vi "Manual_mode.vi"(8 "error in (no error)":errorcluster) -> (0 "error in (out)":errorcluster)   [LabVIEW 2024, in "MANUAL_MODE.lvlib"]
doc: "This template is for the Queued Message Handler design pattern.\n\nThe Event Handling Loop generates messages based on user interface actions.\n\nThe Message Handling Loop processes messages generated by the Event Handling Loop, or by other messages. The messages are string values, so new messages can be added easily to the Message Cases case structure in the Message Handling Loop. Each message cluster can also provide an optional value for Message Data, which is a variant that can be converted to whatever message-specific data is required."
uses:
  MANUAL_MODE.lvlib
  support/FCT_DO_UI.ctl
  support/EOL_DO_UI.ctl
  controls/Manual UI Data.ctl
  PrivateControls/FGV_Queue_Control.ctl
  ADAM_DI/support/Relay_enum_IN.ctl
  <vilib>/Utility/error.llb/Error Cluster From Error Code.vi
  <vilib>/ErrorRing/Error Ring.xnode
  support/Message Queue/Manual Message Queue.lvlib
  support/User Event - Stop/Manual User Event - Stop.lvlib
  Launcher/Launcher_DTU.lvlib
  ADAM_DI/ADAM_DI.lvlib
  Relay_Module/Relay_Module.lvlib
panel:
  in  "Tab Control":T1(tab)
  in  "FCT/EOL":u16(ring) items=["<SELECT>", "FCT", "EOL"]
  in  "Init. INSTR.":bool
  in  "Exit":bool
  in  "DUT":u8=1 min=1 max=10 step=1
  in  "Relay-FCT/EOL":enum32{"FCT", "EOL"}(tab)
  in  "FCT_Relay - OUTPUT":T2
  in  "EOL_Relay - OUTPUT":T3
  out "ADAM_Card - INPUT":T4
  out "queue name 2":string
  out "queue name":string
  out "Display <Replace Me>":string
  # "These controls have associated \"Value Changed\" events configured in the Event Structure on the diagram.\n\nReplace them (and reconfigure the Event Structure) with the controls you need for your application."
  # "This template is for the Queued Message Handler design pattern.\n\nSee the block diagram for more information on how to use this template."
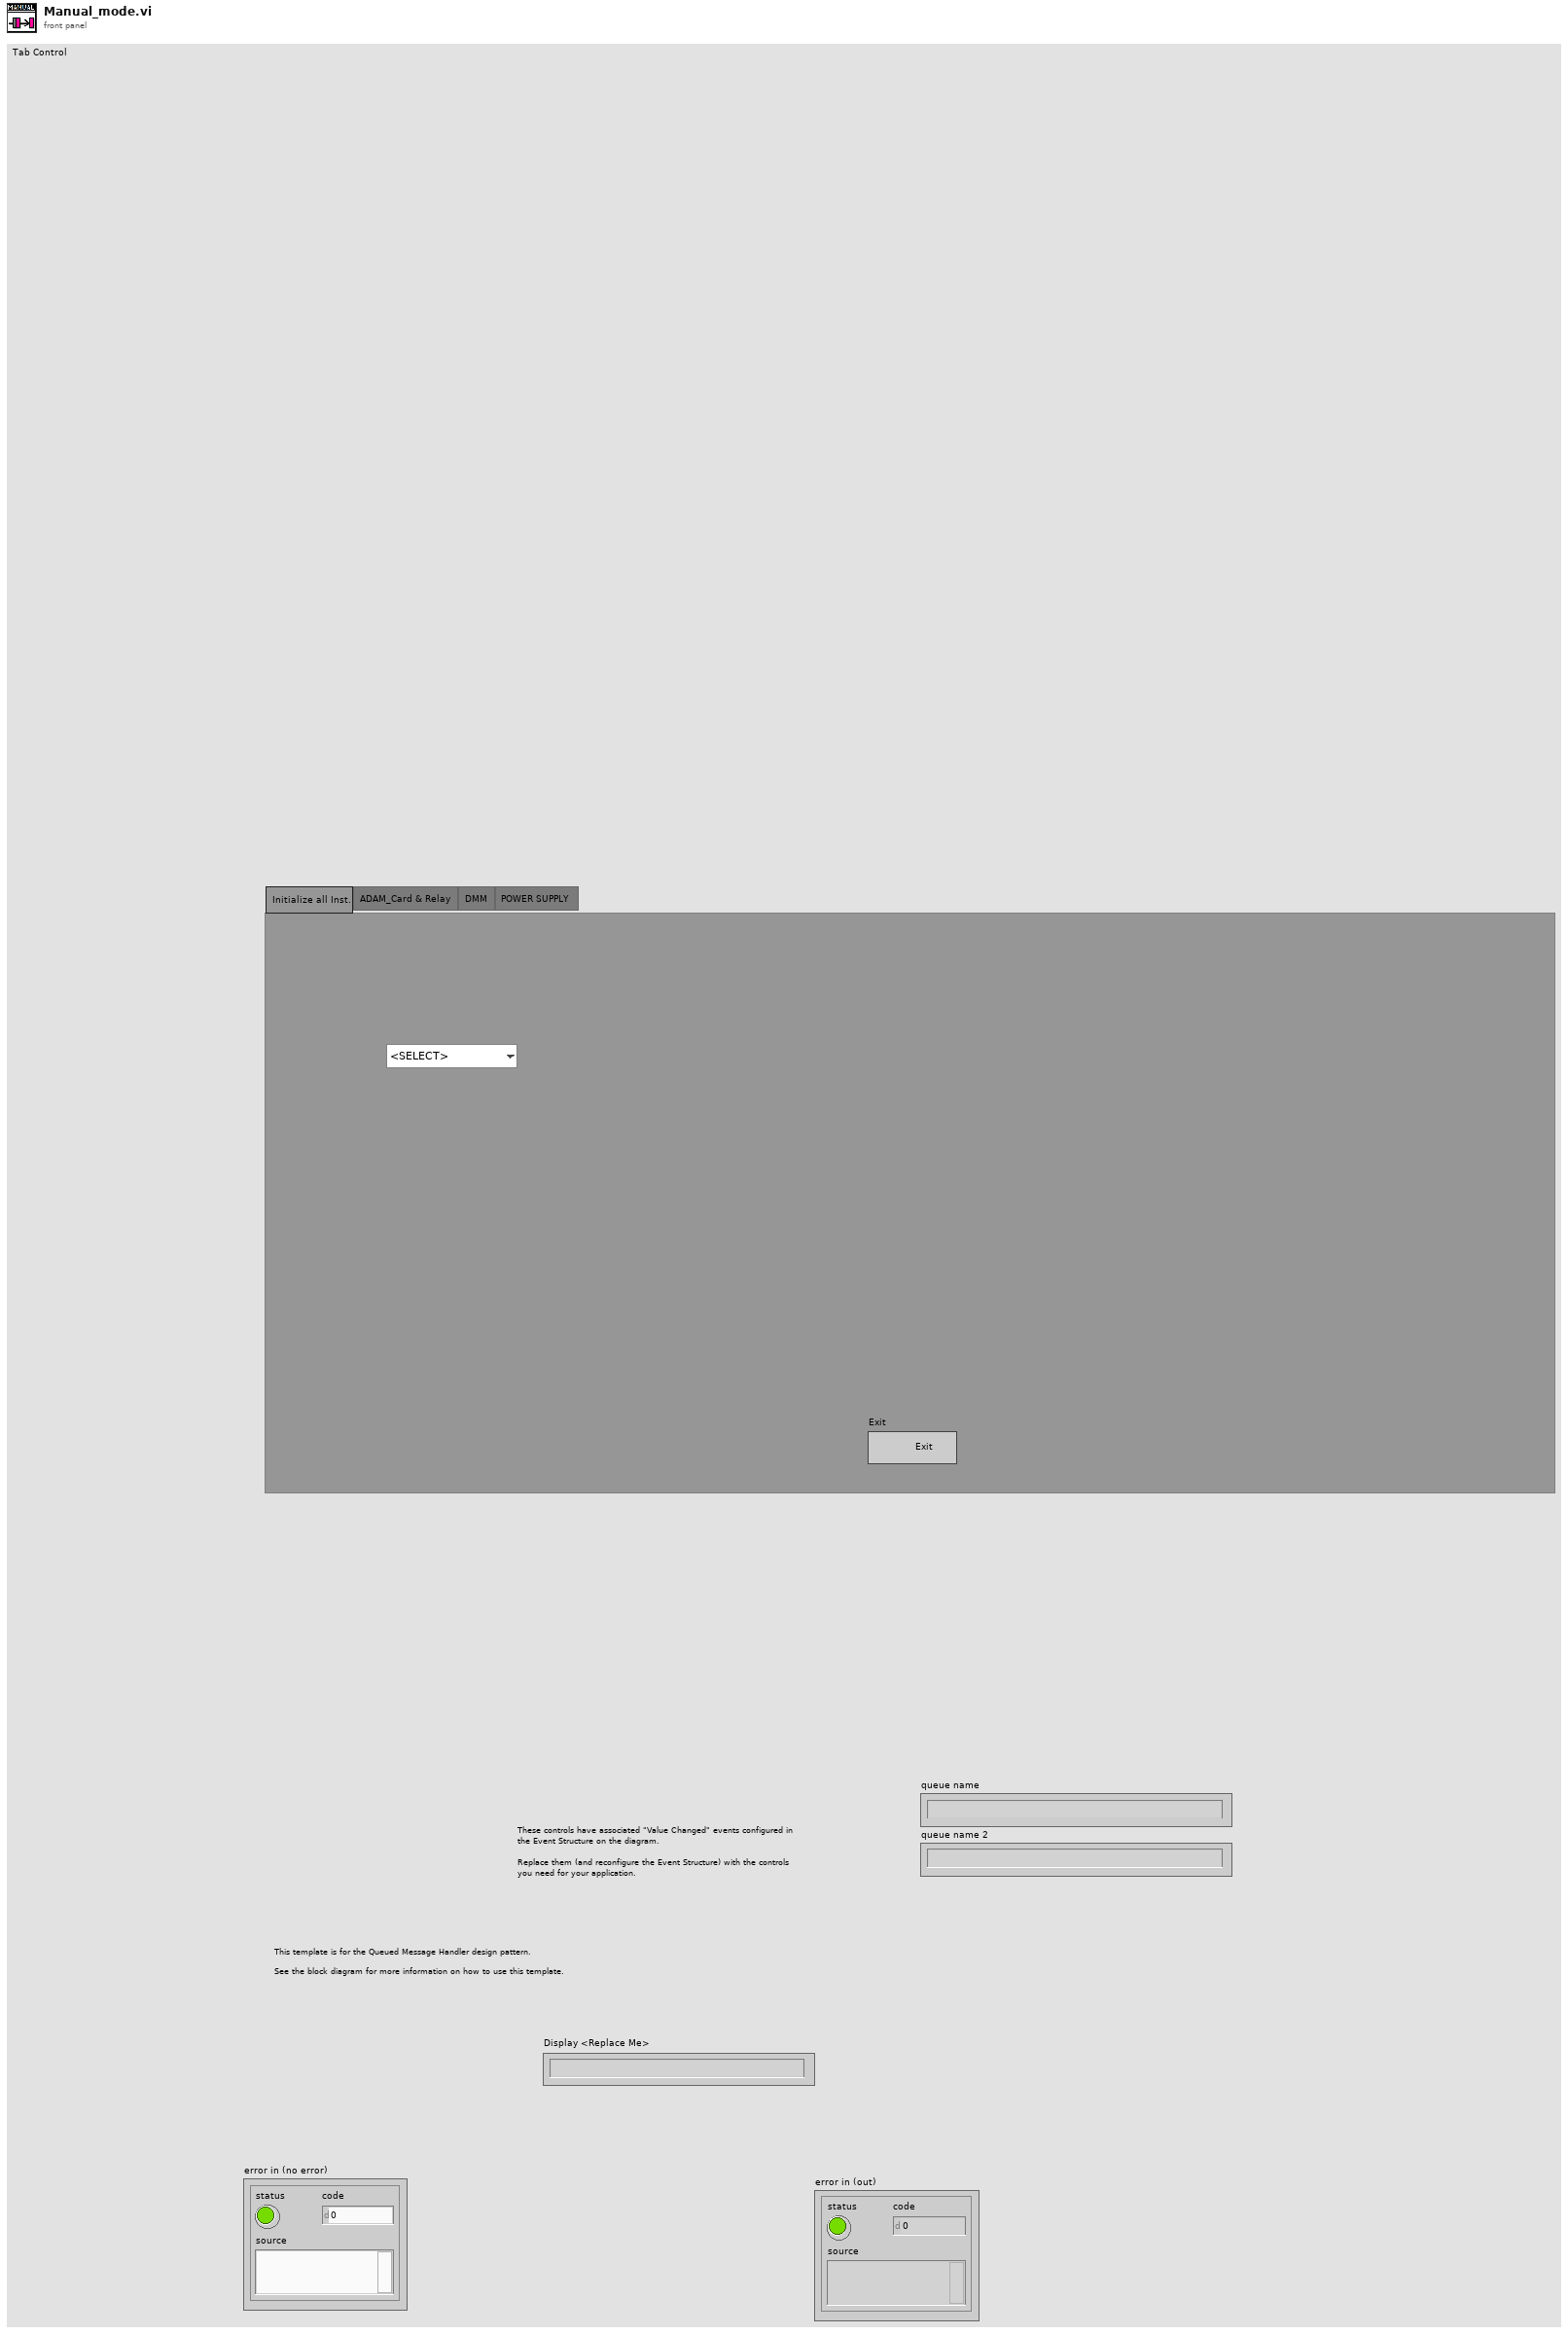
[diagram p1: front panel]
types:
  T1 = enum32{"Initialize all Inst.", "ADAM_Card & Relay", "DMM", "POWER SUPPLY"}
  T2 = typedef "FCT_DO_UI.ctl" = cluster{"CONN_SUPPLY":bool, "HB_CONN":bool, "L_IND_CONN":bool, "R_IND_CONN":bool, "SW1":bool, "SW2":bool, "CAN_H":bool, "CAN_L":bool, "CYLINDER_ON/OFF":bool, "SPARE_1":bool, "SPARE_2":bool, "Tower Red":bool, "Tower Amber":bool, "Tower Green":bool, "Tower Buzzer":bool, "SLIMRELAY_DUT":bool}
  T3 = typedef "EOL_DO_UI.ctl" = cluster{"GND_DMM":bool, "CAN_H_RES":bool, "CAN_L_RES":bool, "L_IND_RES":bool, "R_IND_RES":bool, "HB_CONN_DMM":bool, "14V_RES":bool, "CAN_L_(DMM-)":bool, "CAN_H":bool, "CAN_L":bool, "14V":bool, "GND":bool, "HB_CONN":bool, "L_IND":bool, "R_IND":bool, "CYLINDER_DUT":bool, "CYL_PB_1":bool, "CYL_PB_2":bool, "DUT_PASS":bool, "DUT_FAIL":bool, "SPARE1":bool, "Tower Red_EOL":bool, "Tower Amber_EOL":bool, "Tower Green_EOL":bool, "Tower Buzzer_EOL":bool}
  T4 = cluster{"EMERGENCY":bool, "CONTROL ON":bool, "START DUT 1":bool, "START DUT 2":bool, "STOP DUT 1":bool, "STOP DUT 2":bool, "FCT PPS 1":bool, "FCT PPS 2":bool, "DUT 1 REED CYL UP":bool, "DUT 1 REED CYL DOWN":bool, "DUT 2 REED CYL UP":bool, "DUT 2 REED CYL DOWN":bool, "LIGHT CURTAIN":bool}
  T5 = typedef "MANUAL_MODE.lvlib/FGV_Queue_Control.ctl" = enum16{"Release", "Get", "Set"}
  T6 = typedef "MANUAL_MODE.lvlib/Manual UI Data.ctl" = cluster{"Boolean <Replace Me>":bool, "Status":string, "Numeric <Replace Me>":dbl, "Configuration_Path":path, "Equipment_Combined_Path":path, "Equipment_Common_Path":path, "Equip_List_Common":string[], "Equip_List_Combined":string[], "DTU1_Common-Array_Q":refnum<queue>[], "DTU2_Common-Array_Q":refnum<queue>[], "DTU1_Combined-Array_Q":refnum<queue>[], "DTU2_Combined-Array_Q":refnum<queue>[], "DTU1_Common-Array_N":refnum<notifier>[], "DTU2_Common-Array_N":refnum<notifier>[], "DTU1_Combined-Array_N":refnum<notifier>[], "DTU2_Combined-Array_N":refnum<notifier>[], "ADAM_loop_Q":refnum<queue>, "DUT":u8, "FCT/EOL":u16}
  T7 = typedef "MANUAL_MODE.lvlib/Manual Message Queue.lvlib/All Message Queues.ctl" = cluster{"UI":refnum<queue>, "QSM":refnum<queue>}
  T8 = cluster{"Message":string, "Message Data":variant}
  T9 = enum16{"Read", "Write", "All_sections", "All_values", "Remove key&section"}
  T10 = typedef "Relay_Module.lvlib/Relay_Enum_OUT.ctl" = enum16{"CONN_SUPPLY_%d_FCT", "HB_CONN_%d_FCT", "L_IND_CONN_%d_FCT", "R_IND_CONN_%d_FCT", "SW1_%d_FCT", "SW2_%d_FCT", "CAN_H_%d_FCT", "CAN_L_%d_FCT", "CYLINDER_ON/OFF_%d_FCT", "SPARE_1_%d_FCT", "SPARE_2_%d_FCT", "Tower Red", "Tower Amber", "Tower Green", "Tower Buzzer", "SLIMRELAY_DUT_%d_FCT", "GND_DMM_%d_EOL", "CAN_H_RES_%d_EOL", "CAN_L_RES_%d_EOL", "L_IND_RES_%d_EOL", "R_IND_RES_%d_EOL", "HB_CONN_DMM_%d_EOL", "14V_RES_%d_EOL", "CAN_L_(DMM-)_%d_EOL", "CAN_H_%d_EOL", "CAN_L_%d_EOL", "14V_%d_EOL", "GND_%d_EOL", "HB_CONN_%d_EOL", "L_IND_%d_EOL", "R_IND_%d_EOL", "CYLINDER_DUT_%d_EOL", "CYL_PB_1_%d_EOL", "CYL_PB_2_%d_EOL", "DUT_PASS_%d_EOL", "DUT_FAIL_%d_EOL", "SPARE1_%d_EOL", "Tower Red_EOL", "Tower Amber_EOL", "Tower Green_EOL", "Tower Buzzer_EOL"}
  T11 = typedef "ADAM_DI.lvlib/Relay_enum_IN.ctl" = enum16{"EMERGENCY", "CONTROL ON", "START DUT 1", "START DUT 2", "STOP DUT 1", "STOP DUT 2", "PPS DUT 1", "PPS DUT 2", "REED CYL UP DUT 1", "REED CYL DOWN DUT 1", "REED CYL UP DUT 2", "REED CYL DOWN DUT 2", "LIGHT CURTAIN"}
  T12 = cluster{"DOs_out[0]":bool, "DOs_out[1]":bool, "DOs_out[2]":bool, "DOs_out[3]":bool, "DOs_out[4]":bool, "DOs_out[5]":bool, "DOs_out[6]":bool, "DOs_out[7]":bool, "DOs_out[8]":bool, "DOs_out[9]":bool, "DOs_out[10]":bool, "DOs_out[11]":bool, "DOs_out[12]":bool}
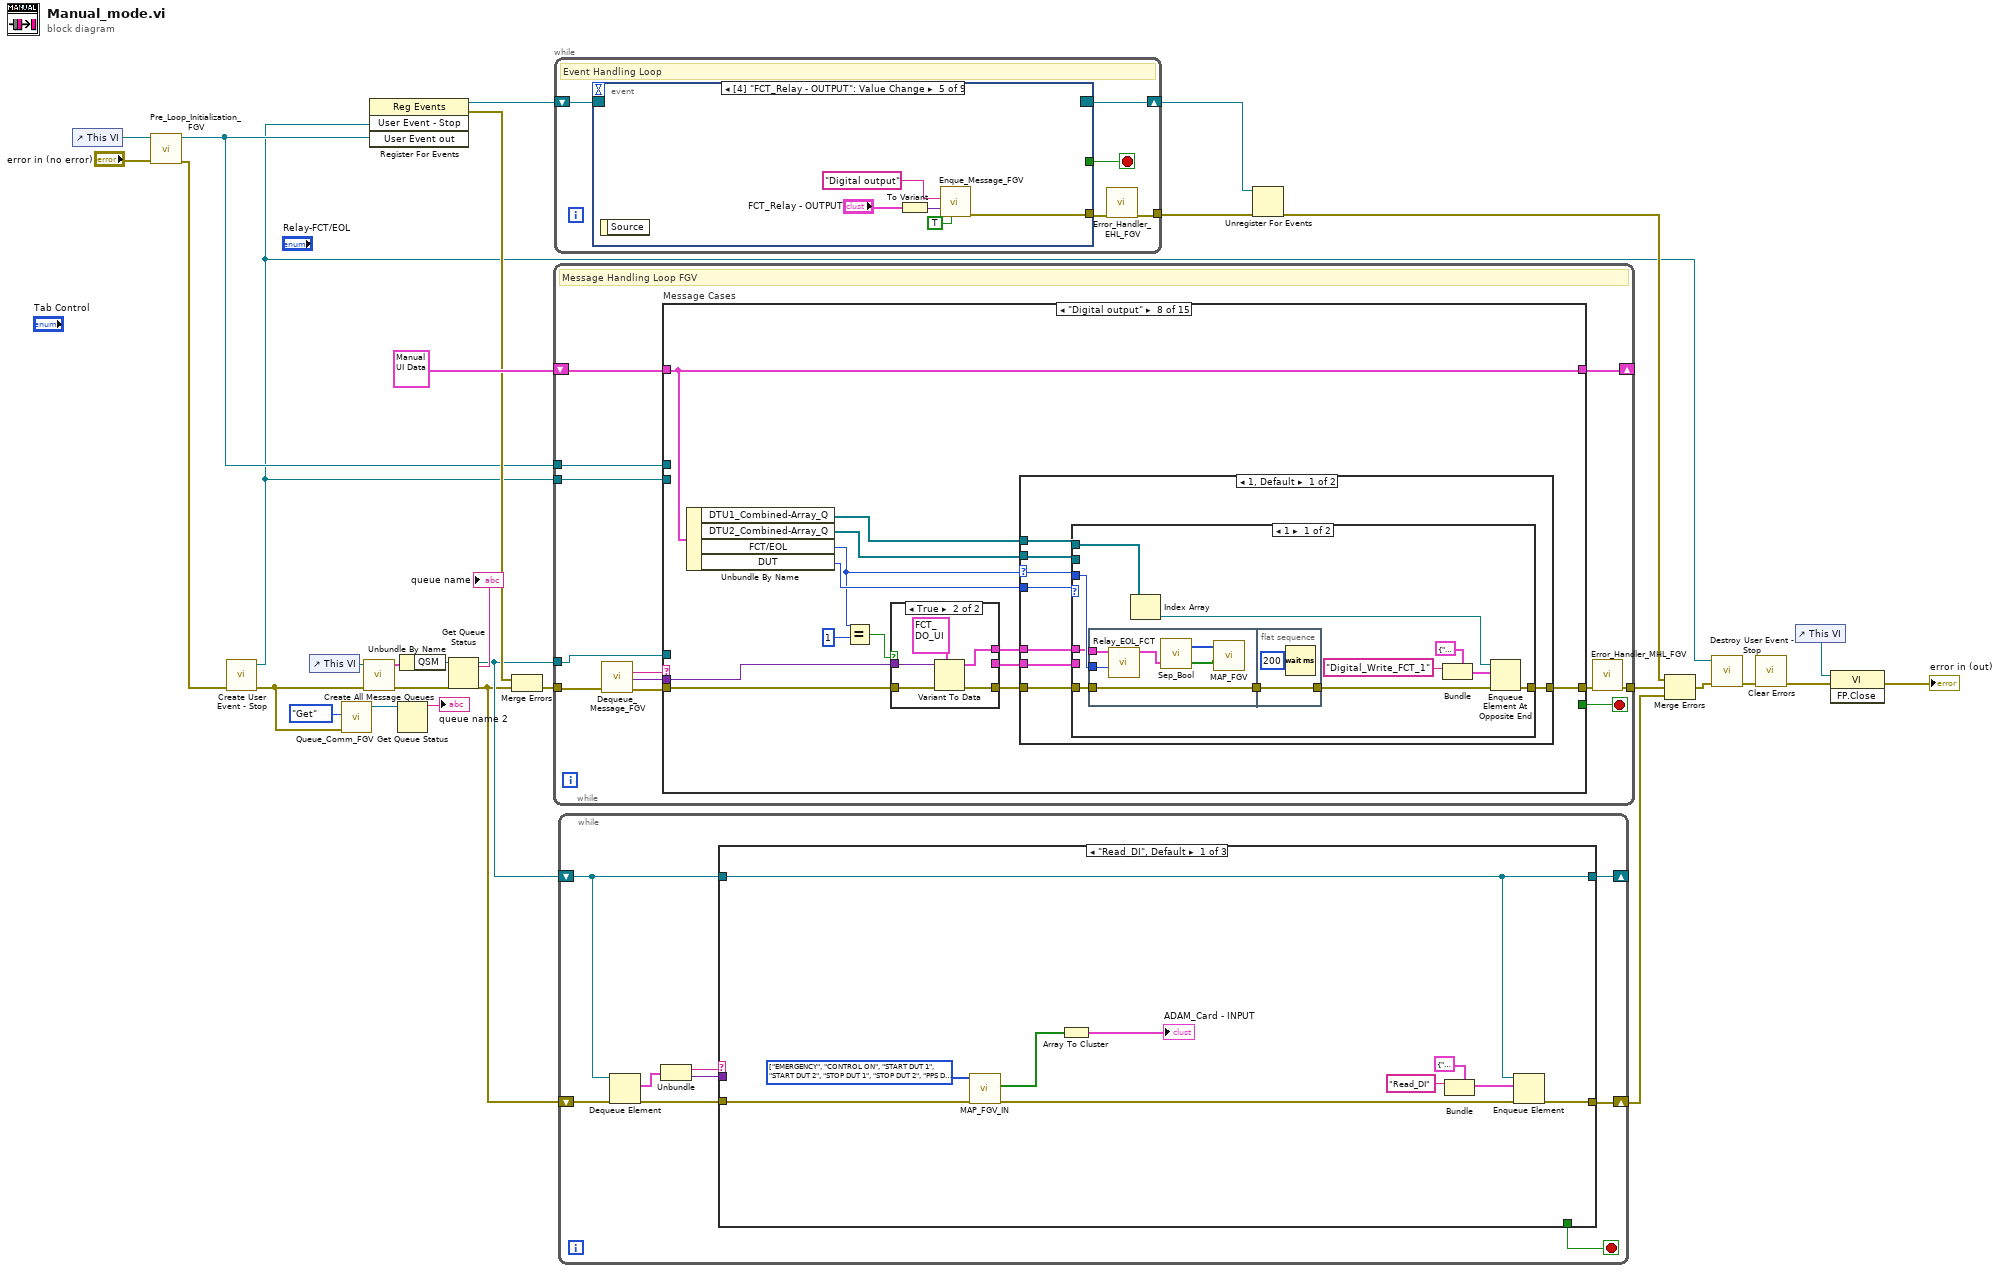
[diagram p0: block diagram]
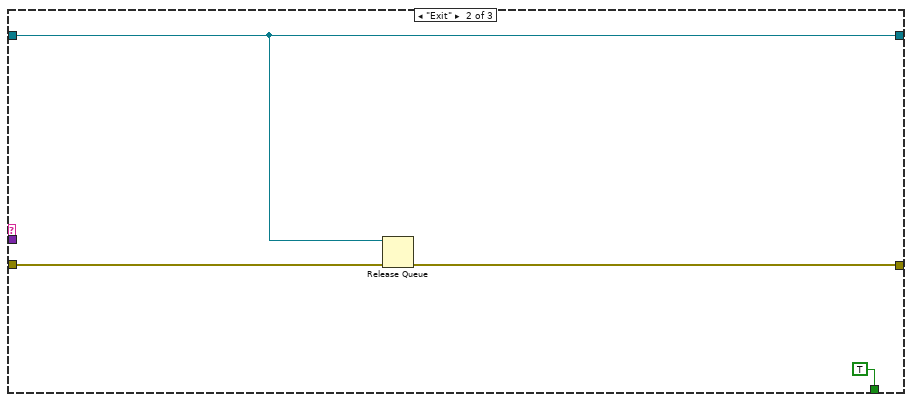
[diagram p2: hidden frame]
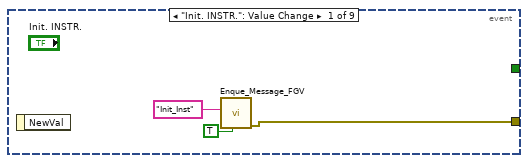
[diagram p4: hidden frame]
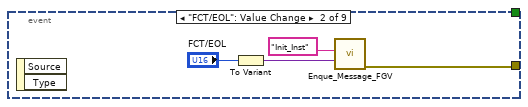
[diagram p5: hidden frame]
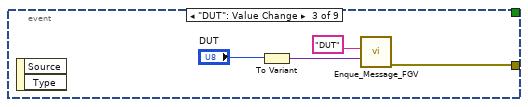
[diagram p6: hidden frame]
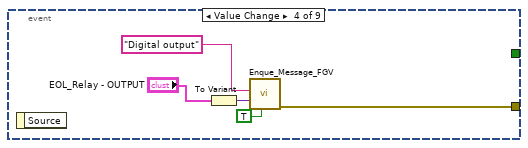
[diagram p7: hidden frame]
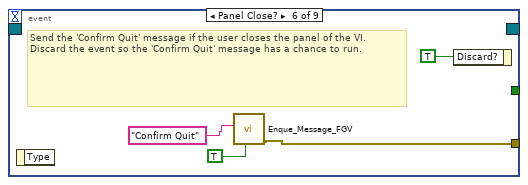
[diagram p8: hidden frame]
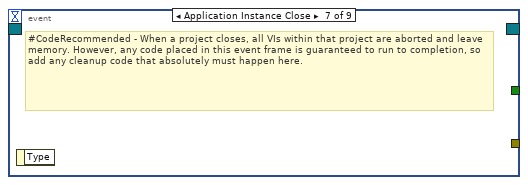
[diagram p9: hidden frame]
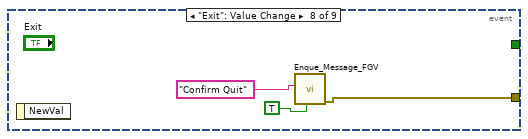
[diagram p10: hidden frame]
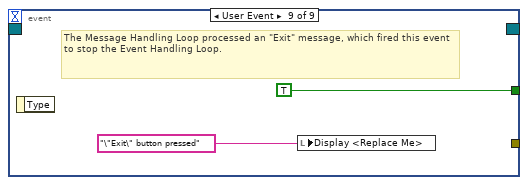
[diagram p11: hidden frame]
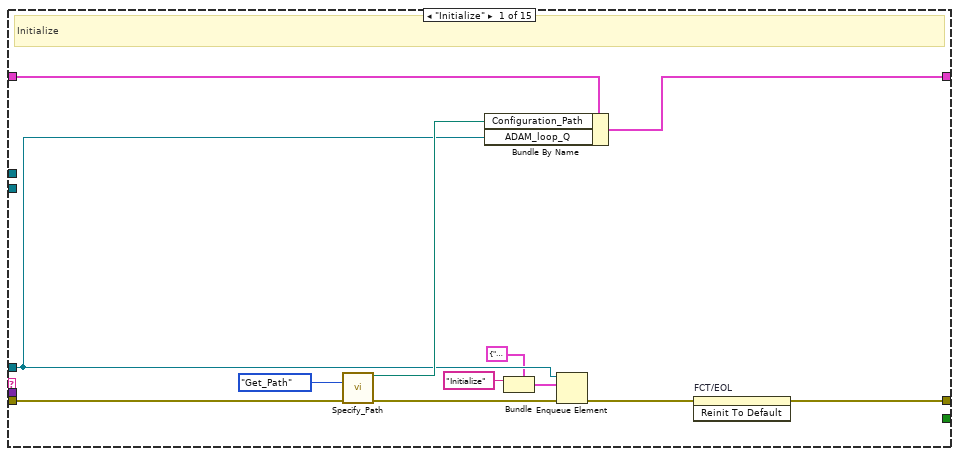
[diagram p12: hidden frame]
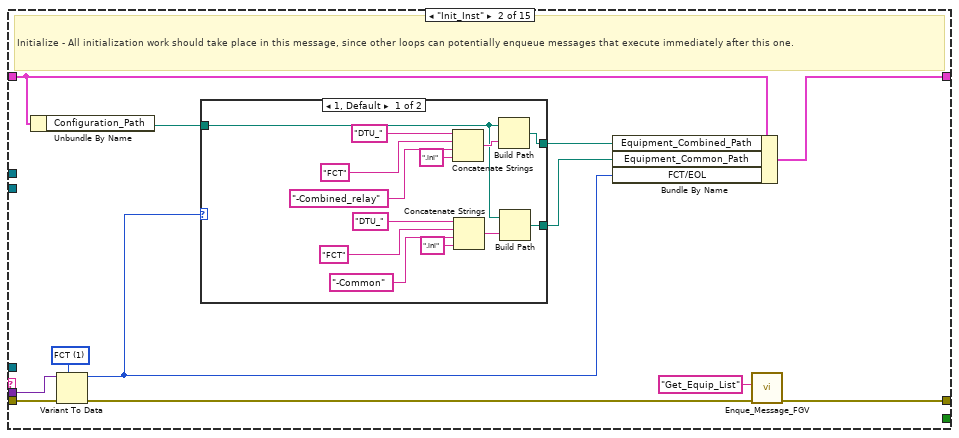
[diagram p13: hidden frame]
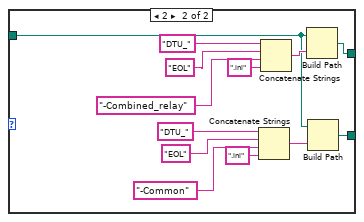
[diagram p14: hidden frame]
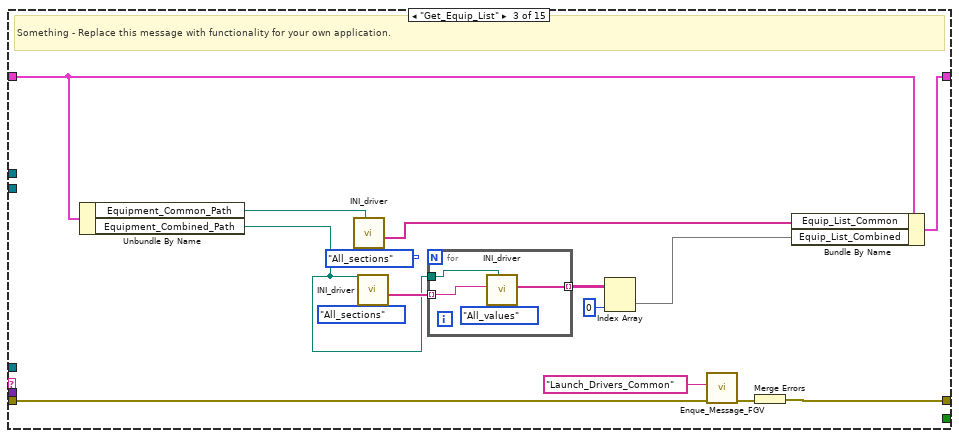
[diagram p15: hidden frame]
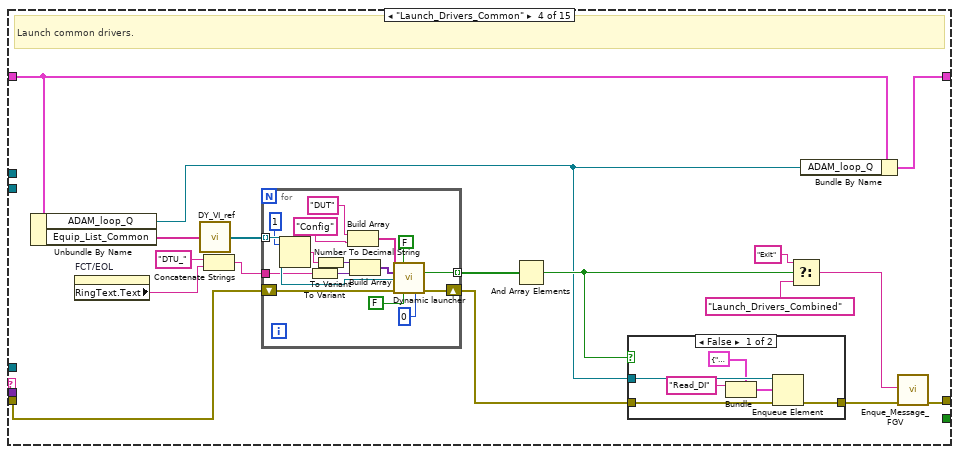
[diagram p16: hidden frame]
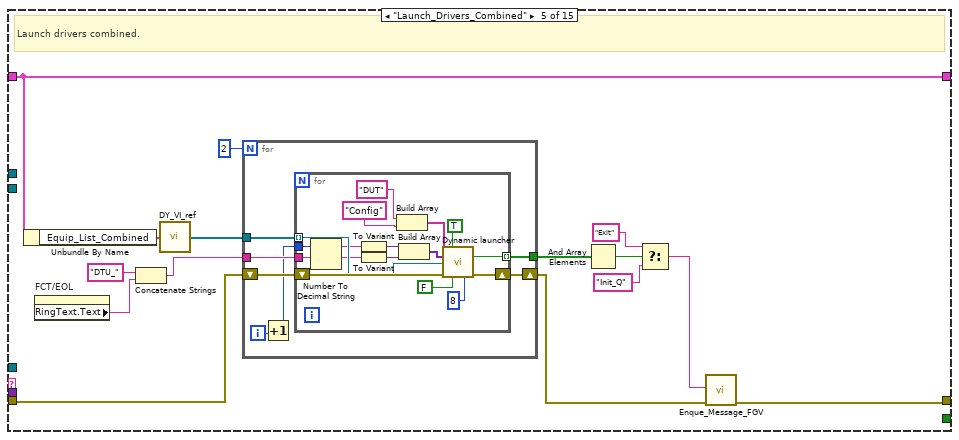
[diagram p18: hidden frame]
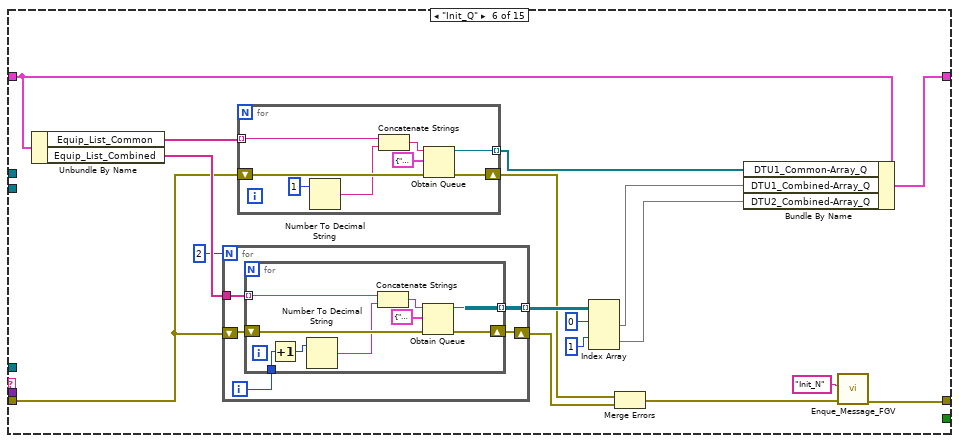
[diagram p19: hidden frame]
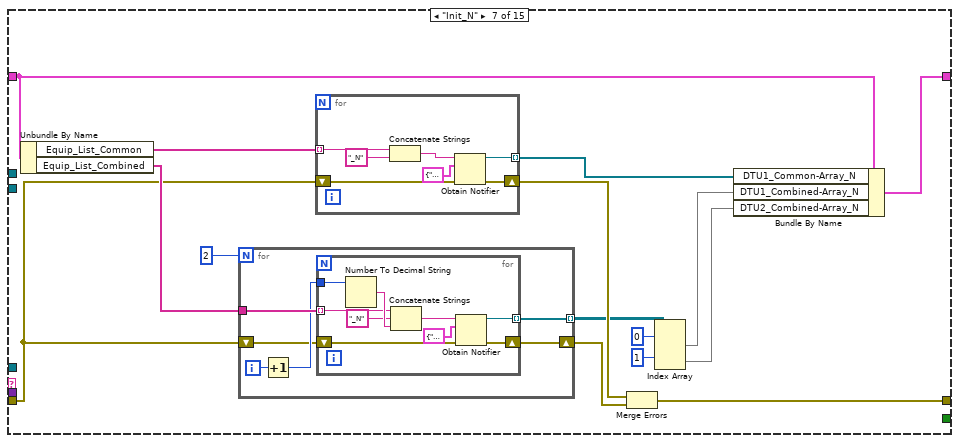
[diagram p20: hidden frame]
diagram:
  n1 = control-ref of="This VI"() -> (w18:refnum<vi>)
  n2 = call "Pre_Loop_Initialization_FGV.vi"("error in (no error)"="error in (no error)", "VI in"=w18) -> ("error out"=w16:errorcluster, "User Event out"=w8:refnum<user-event>)  [unwired: 8 in]
  n3 = call "Create User Event - Stop.vi"("error in (no error)"=w16) -> ("error out"=w12:errorcluster, "User Event - Stop"=w7:refnum<user-event>)  [unwired: 9 in]
  n4 = control-ref of="This VI"() -> (w14:refnum<vi>)
  n5 = call "Queue_Comm_FGV.vi"("error in (no error)"=w12, "Enum"=FGV_Queue_Control."Get") -> ("queue Out"=w10:refnum<queue>)  [unwired: 8 in, 1 out]
  n6 = call "Create All Message Queues.vi"("error in (no error)"=w12, "This VI"=w14) -> ("error out"=w5:errorcluster, "Message Queues out"=w29:T7)  [unwired: 8 in]
  n7 = register-events(w7, w8) -> (reference out=w21:refnum<event-registration>, error out=w19:errorcluster)  [unwired: 2 in]
  n8 = Get Queue Status(queue=w10) -> (queue name=→"queue name 2":string)  [unwired: 2 in, 7 out]
  n9 = Unbundle By Name(w29) -> ("QSM"=w27:refnum<queue>)
  n10 = Get Queue Status(queue=w27) -> (queue out=w6:refnum<queue>, queue name=→"queue name":string)  [unwired: 2 in, 6 out]
  n11 = Merge Errors(w19, w5) -> (w20:errorcluster)
  n12 = while {
    tunnel: w6 -> [w30]
    shift-right: [w40] -> _
    shift-left: T6 {"Boolean <Replace Me>"=FALSE, "Status"="", "Numeric <Replace Me>"=0.0, "Configuration_Path"=path "", "Equipment_Combined_Path"=path "", "Equipment_Common_Path"=path "", "Equip_List_Common"=[], "Equip_List_Combined"=[], "DTU1_Common-Array_Q"=[], "DTU2_Common-Array_Q"=[], "DTU1_Combined-Array_Q"=[], "DTU2_Combined-Array_Q"=[], "DTU1_Common-Array_N"=[], "DTU2_Common-Array_N"=[], "DTU1_Combined-Array_N"=[], "DTU2_Combined-Array_N"=[], "ADAM_loop_Q"=refnum, "DUT"=1, "FCT/EOL"=0} ("Data Cluster") -> [w41]
    tunnel: w8 -> [w38]
    tunnel: w20 -> [w37]
    tunnel: [w32] -> w28
    tunnel: w7 -> [w31]
    stop <- w39 stop-if-true
    # "Message Handling Loop FGV"
    n13 = call "Dequeue_Message_FGV.vi"("error in (no error)"=w37) -> ("error out"=w36:errorcluster, "Message Data"=w35:variant, "Message"=w34:string)  [unwired: 8 in]
    n14 = case "Message Cases" shown="\"Digital output\"" w34 {
      selector: w34 -> [_ _ _ _ _ _ _ _ _ _ _ _ _ _ w499]
      tunnel: w36 -> [w49 w64 w104 w119 w156 w195 w239 w277 w387 w392 w401 w411 w445 w484 _]
      tunnel: [w42 w65 w106 w127 w165 w191 w236 w275 w384 w393 w395 w419 w453 w493 w500] -> w33
      tunnel: w41 -> [w52 w62 w103 w126 w164 w199 w230 w276 w386 w394 w400 w409 w452 w495 w501]
      tunnel: [w51 w59 w102 w115 w164 w198 w229 w276 w385 w394 w400 w409 w452 w495 w501] -> w40
      tunnel: [_ _ _ _ _ _ _ _ _ _ _ _ _ TRUE _] -> w39
      tunnel: w35 -> [_ w57 _ _ _ _ _ w270 w383 w391 w399 _ _ w491 _]
      tunnel: w38 -> [_ _ _ _ _ _ _ _ _ _ _ _ _ w492 _]
      tunnel: w31 -> [_ _ _ _ _ _ _ _ _ _ _ _ _ w488 _]
      tunnel: w30 -> [w47 _ _ _ _ _ _ _ _ _ _ w412 _ _ _]
      frame "Initialize" {
        # "Initialize"
        n15 = call "Specify_Path.vi"("Path_Enum"=enum16{"Find_Path", "Get_Path"}."Get_Path", "error in (no error)"=w49) -> ("Configurations"=w50:path, "error out"=w48:errorcluster)  [unwired: 6 in, 6 out]
        n16 = Bundle By Name(cluster=w52, "Configuration_Path"=w50, "ADAM_loop_Q"=w47) -> (w51:T6)
        n17 = Bundle(cluster=T8 {"Message"="", "Message Data"=variant} ("Message Cluster"), "Message"="Initialize") -> (w45:T8)  [unwired: 1 in]
        n18 = Enqueue Element(queue=w47, element=w45, error in (no error)=w48) -> (error out=w43:errorcluster)  [unwired: 1 in, 2 out]
        n19 = invoke on="FCT/EOL" class="Ring (strict)" method="Reinit To Default"(error in=w43) -> (error out=w42:errorcluster)  [unwired: 2 in, 2 out]
      }
      frame "Init_Inst" {
        w54 = u16 1 items=["<SELECT>", "FCT", "EOL"] ("FCT/EOL")
        # "Initialize - All initialization work should take place in this message, since other loops can potentially enqueue messages that execute immediately after this one."
        n20 = Unbundle By Name(w62) -> ("Configuration_Path"=w63:path)
        n21 = Variant To Data(error in=w64, type=w54, Variant=w57) -> (data=w55:u16, error out=w58:errorcluster)
        n22 = case shown="1, Default" w55 {
          tunnel: w63 -> [w66 w82]
          tunnel: [w68 w81] -> w61
          tunnel: [w67 w80] -> w60
          frame 1, Default {
            n23 = Concatenate Strings("DTU_" ("string"), "FCT" ("regular expression"), "-Combined_relay" ("string"), ".ini" ("string")) -> (w78:string)
            n24 = Concatenate Strings("DTU_" ("string"), "FCT" ("regular expression"), "-Common" ("string"), ".ini" ("string")) -> (w69:string)
            n25 = Build Path(base path=w66, name or relative path=w78) -> (appended path=w68:path)
            n26 = Build Path(base path=w66, name or relative path=w69) -> (appended path=w67:path)
          }
          frame 2 {
            n27 = Concatenate Strings("DTU_" ("string"), "EOL" ("regular expression"), "-Common" ("string"), ".ini" ("string")) -> (w83:string)
            n28 = Concatenate Strings("DTU_" ("string"), "EOL" ("regular expression"), "-Combined_relay" ("string"), ".ini" ("string")) -> (w91:string)
            n29 = Build Path(base path=w82, name or relative path=w91) -> (appended path=w81:path)
            n30 = Build Path(base path=w82, name or relative path=w83) -> (appended path=w80:path)
          }
        }
        n31 = Bundle By Name(cluster=w62, "Equipment_Combined_Path"=w61, "Equipment_Common_Path"=w60, "FCT/EOL"=w55) -> (w59:T6)
        n32 = call "Enque_Message_FGV.vi"("error in (no error)"=w58, "Message"="Get_Equip_List") -> ("error out"=w65:errorcluster)  [unwired: 9 in]
      }
      frame "Get_Equip_List" {
        # "Something - Replace this message with functionality for your own application."
        n33 = Unbundle By Name(w103) -> ("Equipment_Common_Path"=w97:path, "Equipment_Combined_Path"=w96:path)
        n34 = call "INI_driver.vi"("Enum"=T9."All_sections", "instrument file path"=w97) -> ("section names"=w92:string[])  [unwired: 6 in, 3 out]
        n35 = call "INI_driver.vi"("Enum"=T9."All_sections", "instrument file path"=w96) -> ("section names"=w98:string[])  [unwired: 6 in, 3 out]
        n36 = for {
          tunnel: w98 -> [w110] mode=indexing
          tunnel: w96 -> [w109]
          tunnel: [w107] -> w94 mode=indexing
          n37 = call "INI_driver.vi"("Enum"=T9."All_values", "instrument file path"=w109, "Section"=w110) -> ("Values out"=w107:string[])  [unwired: 5 in, 3 out]
        }
        n38 = Index Array(array=w94, index (col)=0 ("disabled index (col)")) -> (element=w93:string[])  [unwired: 1 in]
        n39 = call "Enque_Message_FGV.vi"("error in (no error)"=w104, "Message"="Launch_Drivers_Common") -> ("error out"=w105:errorcluster)  [unwired: 9 in]
        n40 = Merge Errors(w105) -> (w106:errorcluster)
        n41 = Bundle By Name(cluster=w103, "Equip_List_Common"=w92, "Equip_List_Combined"=w93) -> (w102:T6)
      }
      frame "Launch_Drivers_Common" {
        # "Launch common drivers."
        n42 = Unbundle By Name(w126) -> ("ADAM_loop_Q"=w114:refnum<queue>, "Equip_List_Common"=w125:string[])
        n43 = property on="FCT/EOL" class="Ring (strict)"() -> ("RingText.Text"=w112:string)  [unwired: 2 in, 2 out]
        n44 = call "DY_VI_ref.vi"("EQUIP LIST"=w125) -> ("VI_ref"=w124:refnum<vi>[])
        n45 = Concatenate Strings("DTU_", w112) -> (w111:string)
        n46 = for {
          shift-right: [w150] -> w118
          shift-left: w119 -> [w142]
          tunnel: [w149] -> w122 mode=indexing
          tunnel: w124 -> [w138] mode=indexing
          tunnel: w111 -> [w137]
          n47 = Number To Decimal String(number=1) -> (decimal integer string=w135:string)  [unwired: 1 in]
          n48 = To Variant(anything=w137) -> (Variant=w143:variant)
          n49 = To Variant(anything=w135) -> (Variant=w144:variant)
          n50 = Build Array("DUT", "Config") -> (w146:string[])
          n51 = Build Array(w144, w143) -> (w145:variant[])
          n52 = call "Dynamic launcher.vi"("element"=w146, "Clone ?"=FALSE, "Value"=w145, "VI Refnum"=w138, "error in (no error)"=w142, "Open FP"=FALSE, "options"=0) -> ("Failed"=w149:bool, "error out"=w150:errorcluster)  [unwired: 6 in, 1 out]
        }
        n53 = And Array Elements(Boolean array=w122) -> (logical AND=w116:bool)
        n54 = case shown="False" w116 {
          tunnel: w118 -> [w133 w134]
          tunnel: [w132 w134] -> w117
          tunnel: w114 -> [w131 _]
          frame False {
            n55 = Bundle(cluster=T8 {"Message"="", "Message Data"=variant} ("Message Cluster"), "Message"="Read_DI") -> (w128:T8)  [unwired: 1 in]
            n56 = Enqueue Element(queue=w131, element=w128, error in (no error)=w133) -> (error out=w132:errorcluster)  [unwired: 1 in, 2 out]
          }
          frame True {
          }
        }
        n57 = Select(t="Exit" ("f"), s=w116, f="Launch_Drivers_Combined") -> (s? t:f=w120:string)
        n58 = Bundle By Name(cluster=w126, "ADAM_loop_Q"=w114) -> (w115:T6)
        n59 = call "Enque_Message_FGV.vi"("error in (no error)"=w117, "Message"=w120) -> ("error out"=w127:errorcluster)  [unwired: 9 in]
      }
      frame "Launch_Drivers_Combined" {
        # "Launch drivers combined."
        n60 = Unbundle By Name(w164) -> ("Equip_List_Combined"=w163:string[])
        n61 = property on="FCT/EOL" class="Ring (strict)"() -> ("RingText.Text"=w152:string)  [unwired: 2 in, 2 out]
        n62 = Concatenate Strings("DTU_", w152) -> (w151:string)
        n63 = call "DY_VI_ref.vi"("EQUIP LIST"=w163) -> ("VI_ref"=w162:refnum<vi>[])
        n64 = for {
          N: 2 -> [_]
          tunnel: w162 -> [w172]
          tunnel: [w171] -> w159
          shift-right: [w169] -> w155
          shift-left: w156 -> [w170]
          tunnel: w151 -> [w167]
          i -> [w168]
          n65 = Increment(x=w168) -> (x+1=w166:i32)
          n66 = for {
            shift-right: [w188] -> w169
            shift-left: w170 -> [w180]
            tunnel: [w187] -> w171 mode=indexing
            tunnel: w172 -> [w176] mode=indexing
            tunnel: w166 -> [w175]
            tunnel: w167 -> [w174]
            n67 = Number To Decimal String(number=w175) -> (decimal integer string=w173:string)  [unwired: 1 in]
            n68 = To Variant(anything=w173) -> (Variant=w182:variant)
            n69 = To Variant(anything=w174) -> (Variant=w181:variant)
            n70 = Build Array("DUT", "Config") -> (w184:string[])
            n71 = Build Array(w182, w181) -> (w183:variant[])
            n72 = call "Dynamic launcher.vi"("element"=w184, "Clone ?"=TRUE, "Value"=w183, "VI Refnum"=w176, "error in (no error)"=w180, "Open FP"=FALSE, "options"=8) -> ("Failed"=w187:bool, "error out"=w188:errorcluster)  [unwired: 6 in, 1 out]
          }
        }
        n73 = And Array Elements(Boolean array=w159) -> (logical AND=w160:bool)
        n74 = Select(t="Exit" ("f"), s=w160, f="Init_Q") -> (s? t:f=w157:string)
        n75 = call "Enque_Message_FGV.vi"("error in (no error)"=w155, "Message"=w157) -> ("error out"=w165:errorcluster)  [unwired: 9 in]
      }
      frame "Init_Q" {
        n76 = Unbundle By Name(w199) -> ("Equip_List_Common"=w205:string[], "Equip_List_Combined"=w204:string[])
        n77 = for {
          N: 2 -> [_]
          tunnel: w204 -> [w218]
          tunnel: [w216] -> w201 mode=indexing
          shift-right: [w214] -> w193
          shift-left: w195 -> [w215]
          i -> [w217]
          n78 = for {
            shift-right: [w226] -> w214
            shift-left: w215 -> [w227]
            tunnel: w218 -> [w223] mode=indexing
            tunnel: [w222] -> w216 mode=indexing
            tunnel: w217 -> [w219]
            n79 = Increment(x=w219) -> (x+1=w220:i32)
            n80 = Number To Decimal String(number=w220) -> (decimal integer string=w221:string)  [unwired: 1 in]
            n81 = Concatenate Strings(w223, w221) -> (w224:string)
            n82 = Obtain Queue(name (unnamed)=w224, element data type=T8 {"Message"="", "Message Data"=variant} ("element"), error in (no error)=w227) -> (queue out=w222:refnum<queue>, error out=w226:errorcluster)  [unwired: 2 in, 1 out]
          }
        }
        n83 = for {
          shift-right: [w212] -> w194
          shift-left: w195 -> [w213]
          tunnel: w205 -> [w209] mode=indexing
          tunnel: [w208] -> w189 mode=indexing
          n84 = Number To Decimal String(number=1) -> (decimal integer string=w207:string)  [unwired: 1 in]
          n85 = Concatenate Strings(w209, w207) -> (w210:string)
          n86 = Obtain Queue(name (unnamed)=w210, element data type=T8 {"Message"="", "Message Data"=variant} ("element"), error in (no error)=w213) -> (queue out=w208:refnum<queue>, error out=w212:errorcluster)  [unwired: 2 in, 1 out]
        }
        n87 = Index Array(array=w201, index (row) #1=0 ("index (row)"), index (row) #2=1 ("index (row)")) -> (element #1=w197:refnum<queue>[], element #2=w196:refnum<queue>[])  [unwired: 2 in]
        n88 = Merge Errors(w194, w193) -> (w192:errorcluster)
        n89 = Bundle By Name(cluster=w199, "DTU1_Common-Array_Q"=w189, "DTU1_Combined-Array_Q"=w197, "DTU2_Combined-Array_Q"=w196) -> (w198:T6)
        n90 = call "Enque_Message_FGV.vi"("error in (no error)"=w192, "Message"="Init_N" ("f")) -> ("error out"=w191:errorcluster)  [unwired: 9 in]
      }
      frame "Init_N" {
        n91 = Unbundle By Name(w230) -> ("Equip_List_Common"=w242:string[], "Equip_List_Combined"=w241:string[])
        n92 = for {
          N: 2 -> [_]
          tunnel: w241 -> [w254]
          tunnel: [w252] -> w231 mode=indexing
          shift-right: [w250] -> w237
          shift-left: w239 -> [w251]
          i -> [w255]
          n93 = Increment(x=w255) -> (x+1=w253:i32)
          n94 = for {
            shift-right: [w263] -> w250
            shift-left: w251 -> [w264]
            tunnel: w254 -> [w257] mode=indexing
            tunnel: w253 -> [w262]
            tunnel: [w259] -> w252 mode=indexing
            n95 = Number To Decimal String(number=w262) -> (decimal integer string=w260:string)  [unwired: 1 in]
            n96 = Concatenate Strings(w257, "_N" ("string"), w260) -> (w261:string)
            n97 = Obtain Notifier(name (unnamed)=w261, notification data type=T8 {"Message"="", "Message Data"=variant} ("notification"), error in (no error)=w264) -> (notifier out=w259:refnum<notifier>, error out=w263:errorcluster)  [unwired: 1 in, 1 out]
          }
        }
        n98 = for {
          shift-right: [w248] -> w238
          shift-left: w239 -> [w249]
          tunnel: w242 -> [w244] mode=indexing
          tunnel: [w246] -> w228 mode=indexing
          n99 = Concatenate Strings(w244, "_N" ("string")) -> (w247:string)
          n100 = Obtain Notifier(name (unnamed)=w247, notification data type=T8 {"Message"="", "Message Data"=variant} ("notification"), error in (no error)=w249) -> (notifier out=w246:refnum<notifier>, error out=w248:errorcluster)  [unwired: 1 in, 1 out]
        }
        n101 = Merge Errors(w238, w237) -> (w236:errorcluster)
        n102 = Index Array(array=w231, index (row) #1=0 ("index (row)"), index (row) #2=1 ("index (row)")) -> (element #1=w233:refnum<notifier>[], element #2=w232:refnum<notifier>[])  [unwired: 2 in]
        n103 = Bundle By Name(cluster=w230, "DTU1_Common-Array_N"=w228, "DTU1_Combined-Array_N"=w233, "DTU2_Combined-Array_N"=w232) -> (w229:T6)
      }
      frame "Digital output" {
        n104 = Unbundle By Name(w276) -> ("DTU1_Combined-Array_Q"=w273:refnum<queue>[], "DTU2_Combined-Array_Q"=w272:refnum<queue>[], "FCT/EOL"=w268:u16, "DUT"=w274:u8)
        n105 = Equal?(x=w268, y=u16 1 ("FCT/EOL")) -> (x = y?=w267:bool)
        n106 = case shown="True" w267 {
          tunnel: w277 -> [w282 w287]
          tunnel: [w281 w286] -> w271
          tunnel: w270 -> [w279 w285]
          tunnel: [w278 _] -> w269
          tunnel: [_ w283] -> w266
          frame False {
            n107 = Variant To Data(error in=w282, type=T3 {"GND_DMM"=FALSE, "CAN_H_RES"=FALSE, "CAN_L_RES"=FALSE, "L_IND_RES"=FALSE, "R_IND_RES"=FALSE, "HB_CONN_DMM"=FALSE, "14V_RES"=FALSE, "CAN_L_(DMM-)"=FALSE, "CAN_H"=FALSE, "CAN_L"=FALSE, "14V"=FALSE, "GND"=FALSE, "HB_CONN"=FALSE, "L_IND"=FALSE, "R_IND"=FALSE, "CYLINDER_DUT"=FALSE, "CYL_PB_1"=FALSE, "CYL_PB_2"=FALSE, "DUT_PASS"=FALSE, "DUT_FAIL"=FALSE, "SPARE1"=FALSE, "Tower Red_EOL"=FALSE, "Tower Amber_EOL"=FALSE, "Tower Green_EOL"=FALSE, "Tower Buzzer_EOL"=FALSE} ("EOL_Relay - OUTPUT"), Variant=w279) -> (data=w278:T3, error out=w281:errorcluster)
          }
          frame True {
            n108 = Variant To Data(error in=w287, type=T2 {"CONN_SUPPLY"=FALSE, "HB_CONN"=FALSE, "L_IND_CONN"=FALSE, "R_IND_CONN"=FALSE, "SW1"=FALSE, "SW2"=FALSE, "CAN_H"=FALSE, "CAN_L"=FALSE, "CYLINDER_ON/OFF"=FALSE, "SPARE_1"=FALSE, "SPARE_2"=FALSE, "Tower Red"=FALSE, "Tower Amber"=FALSE, "Tower Green"=FALSE, "Tower Buzzer"=FALSE, "SLIMRELAY_DUT"=FALSE} ("FCT_Relay - OUTPUT"), Variant=w285) -> (data=w283:T2, error out=w286:errorcluster)
          }
        }
        n109 = case shown="1, Default" w268 {
          selector: w268 -> [w288 w336]
          tunnel: w271 -> [w295 w341]
          tunnel: [w294 w340] -> w275
          tunnel: w274 -> [w291 w339]
          tunnel: w273 -> [w293 w337]
          tunnel: w272 -> [w292 w338]
          tunnel: w269 -> [w290 w335]
          tunnel: w266 -> [w289 _]
          frame 1, Default {
            n110 = case shown="1" w291 {
              tunnel: w295 -> [w298 w317]
              tunnel: [w306 w326] -> w294
              tunnel: w293 -> [w304 _]
              tunnel: w292 -> [_ w324]
              tunnel: w290 -> [_ _]
              tunnel: w289 -> [w299 w320]
              tunnel: w288 -> [w300 w319]
              frame 1 {
                n111 = flat-sequence {
                  tunnel: w300 -> [w312]
                  tunnel: w299 -> [w311]
                  tunnel: w298 -> [w307]
                  tunnel: [w307] -> w296
                  tunnel: [w314] -> w297
                  tunnel: w296 -> [w314]
                  frame #0 {
                    n112 = call "Relay_EOL_FCT.vi"("FCT/EOL"=w312, "FCT_Relay - OUTPUT"=w311) -> ("output cluster"=w310:cluster{cluster{bool, "OUTPUT_CH_Relay":T10}[]})  [unwired: 9 in]
                    n113 = call "Sep_Bool.vi"("output cluster"=w310) -> ("DO_Bool"=w308:bool[], "Array"=w309:T10[])  [unwired: 1 in]
                    n114 = call "MAP_FGV.vi"("DOs"=w308, "Relay_Channel_Out"=w309) -> ()  [unwired: 7 in, 3 out]
                  }
                  frame #1 {
                    n115 = Wait (ms)(milliseconds to wait=u32 200) -> ()  [unwired: 1 out]
                  }
                }
                n116 = Index Array(array=w304) -> (element=w305:refnum<queue>)  [unwired: 1 in]
                n117 = Bundle(cluster=T8 {"Message"="", "Message Data"=variant} ("element"), "Message"="Digital_Write_FCT_1") -> (w302:T8)  [unwired: 1 in]
                n118 = Enqueue Element At Opposite End(queue=w305, element=w302, error in (no error)=w297) -> (error out=w306:errorcluster)  [unwired: 1 in, 2 out]
              }
              frame 2, Default {
                n119 = flat-sequence {
                  tunnel: w320 -> [w332]
                  tunnel: w319 -> [w331]
                  tunnel: w317 -> [w327]
                  tunnel: [w327] -> w315
                  tunnel: [w334] -> w316
                  tunnel: w315 -> [w334]
                  frame #0 {
                    n120 = call "Relay_EOL_FCT.vi"("FCT/EOL"=w331, "FCT_Relay - OUTPUT"=w332) -> ("output cluster"=w330:cluster{cluster{bool, "OUTPUT_CH_Relay":T10}[]})  [unwired: 9 in]
                    n121 = call "Sep_Bool.vi"("output cluster"=w330) -> ("DO_Bool"=w328:bool[], "Array"=w329:T10[])  [unwired: 1 in]
                    n122 = call "MAP_FGV_2.vi"("DOs"=w328, "Relay_Channel_Out"=w329) -> ()  [unwired: 7 in, 3 out]
                  }
                  frame #1 {
                    n123 = Wait (ms)(milliseconds to wait=u32 250) -> ()  [unwired: 1 out]
                  }
                }
                n124 = Index Array(array=w324, index=0) -> (element=w325:refnum<queue>)
                n125 = Bundle(cluster=T8 {"Message"="", "Message Data"=variant} ("element"), "Message"="Digital_Write_FCT_2") -> (w322:T8)  [unwired: 1 in]
                n126 = Enqueue Element At Opposite End(queue=w325, element=w322, error in (no error)=w316) -> (error out=w326:errorcluster)  [unwired: 1 in, 2 out]
              }
            }
          }
          frame 2 {
            n127 = case shown="1" w339 {
              tunnel: w341 -> [w344 w363]
              tunnel: [w352 w372] -> w340
              tunnel: w338 -> [_ w370]
              tunnel: w337 -> [w351 _]
              tunnel: w336 -> [w347 w366]
              tunnel: w335 -> [w346 w365]
              frame 1 {
                n128 = flat-sequence {
                  tunnel: w347 -> [w358]
                  tunnel: w346 -> [w357]
                  tunnel: w344 -> [w353]
                  tunnel: [w353] -> w342
                  tunnel: [w360] -> w343
                  tunnel: w342 -> [w360]
                  frame #0 {
                    n129 = call "Relay_EOL_FCT.vi"("FCT/EOL"=w358, "EOL_Relay - OUTPUT"=w357) -> ("output cluster"=w356:cluster{cluster{bool, "OUTPUT_CH_Relay":T10}[]})  [unwired: 9 in]
                    n130 = call "Sep_Bool_EOL.vi"("output cluster"=w356) -> ("DO_Bool"=w355:bool[], "Array"=w354:T10[])  [unwired: 1 in]
                    n131 = call "MAP_FGV_EOL_1.vi"("DOs"=w355, "Relay_Channel_Out"=w354) -> ()  [unwired: 7 in, 3 out]
                  }
                  frame #1 {
                    n132 = Wait (ms)(milliseconds to wait=u32 250) -> ()  [unwired: 1 out]
                  }
                }
                n133 = Index Array(array=w351) -> (element=w350:refnum<queue>)  [unwired: 1 in]
                n134 = Bundle(cluster=T8 {"Message"="", "Message Data"=variant} ("element"), "Message"="Digital_Write_EOL_1") -> (w349:T8)  [unwired: 1 in]
                n135 = Enqueue Element At Opposite End(queue=w350, element=w349, error in (no error)=w343) -> (error out=w352:errorcluster)  [unwired: 1 in, 2 out]
              }
              frame 2, Default {
                n136 = flat-sequence {
                  tunnel: w366 -> [w378]
                  tunnel: w365 -> [w377]
                  tunnel: w363 -> [w373]
                  tunnel: [w373] -> w361
                  tunnel: [w380] -> w362
                  tunnel: w361 -> [w380]
                  frame #0 {
                    n137 = call "Relay_EOL_FCT.vi"("FCT/EOL"=w378, "EOL_Relay - OUTPUT"=w377) -> ("output cluster"=w376:cluster{cluster{bool, "OUTPUT_CH_Relay":T10}[]})  [unwired: 9 in]
                    n138 = call "Sep_Bool_EOL.vi"("output cluster"=w376) -> ("DO_Bool"=w374:bool[], "Array"=w375:T10[])  [unwired: 1 in]
                    n139 = call "MAP_FGV_EOL_2.vi"("DOs"=w374, "Relay_Channel_Out"=w375) -> ()  [unwired: 7 in, 3 out]
                  }
                  frame #1 {
                    n140 = Wait (ms)(milliseconds to wait=u32 250) -> ()  [unwired: 1 out]
                  }
                }
                n141 = Index Array(array=w370, index=0) -> (element=w371:refnum<queue>)
                n142 = Bundle(cluster=T8 {"Message"="", "Message Data"=variant} ("element"), "Message"="Digital_Write_EOL_2") -> (w368:T8)  [unwired: 1 in]
                n143 = Enqueue Element At Opposite End(queue=w371, element=w368, error in (no error)=w362) -> (error out=w372:errorcluster)  [unwired: 1 in, 2 out]
              }
            }
          }
        }
      }
      frame "DUT" {
        n144 = Variant To Data(error in=w387, type=u8 1 ("DUT"), Variant=w383) -> (data=w381:u8, error out=w384:errorcluster)
        n145 = Bundle By Name(cluster=w386, "DUT"=w381) -> (w385:T6)
      }
      frame "Update Display" {
        # "Update Display - Convert the message data to a string to display in the Data Display indicator."
        n146 = Variant To Data(error in=w392, type="", Variant=w391) -> (data=→"Display <Replace Me>":string, error out=w389:errorcluster)
        n147 = Merge Errors(w389) -> (w393:errorcluster)
      }
      frame "Error" {
        # "#CodeRecommended - If you ever change the name of this \"Error\" message, you'll need to update the name in the Check Loop Error.vi as well."
        # "#CodeRecommended - Consider creating a system for logging errors in some way. These errors are for notification purposes only. Handling of specific errors should be performed in the message frames that generated the error."
        # "Error - Display an error dialog. This message is sent by the \"Error Handler\" VIs at the end of other loops in this application."
        n148 = Variant To Data(error in=w401, type=errorcluster {"status"=FALSE, "code"=0, "source"=""} ("error constant"), Variant=w399) -> (data=w397:errorcluster, error out=w396:errorcluster)
        n149 = call <vilib>:"Simple Error Handler.vi"("error in (no error)"=w397) -> ()  [unwired: 4 in, 5 out]
        n150 = Merge Errors(w396) -> (w395:errorcluster)
      }
      frame "Confirm Quit" {
        # "Confirm Quit - Message that can confirm whether or not the user wants to exit the application."
        n151 = Unbundle By Name(w409) -> ("DTU1_Combined-Array_Q"=w403:refnum<queue>[], "DTU2_Combined-Array_Q"=w402:refnum<queue>[], "DTU1_Common-Array_Q"=w405:refnum<queue>[])
        n152 = Bundle(cluster=T8 {"Message"="", "Message Data"=variant} ("Message Cluster"), "Message"="Exit") -> (w413:T8)  [unwired: 1 in]
        n153 = Enqueue Element(queue=w412, element=w413, error in (no error)=w411) -> (error out=w410:errorcluster)  [unwired: 1 in, 2 out]
        n154 = call <vilib>:"Clear Errors.vi"("error in (no error)"=w410) -> ("error out"=w408:errorcluster)  [unwired: 5 in, 1 out]
        n155 = for {
          shift-right: [w436] -> w407
          shift-left: w408 -> [w437]
          tunnel: w405 -> [w435] mode=indexing
          n156 = Bundle(cluster=T8 {"Message"="", "Message Data"=variant} ("Message Cluster"), "Message"="Exit") -> (w432:T8)  [unwired: 1 in]
          n157 = Enqueue Element(queue=w435, element=w432, error in (no error)=w437) -> (error out=w436:errorcluster)  [unwired: 1 in, 2 out]
        }
        n158 = call <vilib>:"Clear Errors.vi"("error in (no error)"=w407) -> ("error out"=w404:errorcluster)  [unwired: 5 in, 1 out]
        n159 = for {
          shift-right: [w424] -> _
          shift-left: w404 -> [w425]
          tunnel: w403 -> [w423] mode=indexing
          n160 = Bundle(cluster=T8 {"Message"="", "Message Data"=variant} ("Message Cluster"), "Message"="Exit") -> (w420:T8)  [unwired: 1 in]
          n161 = Enqueue Element At Opposite End(queue=w423, element=w420, error in (no error)=w425) -> (error out=w424:errorcluster)  [unwired: 1 in, 2 out]
        }
        n162 = for {
          shift-right: [w430] -> w406
          shift-left: w404 -> [w431]
          tunnel: w402 -> [w429] mode=indexing
          n163 = Bundle(cluster=T8 {"Message"="", "Message Data"=variant} ("Message Cluster"), "Message"="Exit") -> (w426:T8)  [unwired: 1 in]
          n164 = Enqueue Element At Opposite End(queue=w429, element=w426, error in (no error)=w431) -> (error out=w430:errorcluster)  [unwired: 1 in, 2 out]
        }
        n165 = call "Enque_Message_FGV.vi"("Priority"=TRUE ("Priority Message? (F)"), "error in (no error)"=w406, "Message"="Quit2") -> ("error out"=w418:errorcluster)  [unwired: 8 in]
        n166 = Merge Errors(w418) -> (w419:errorcluster)
      }
      frame "Quit2" {
        # "Duplicate this frame when creating new messages.  Change this comment in the duplicated frame to describe this message."
        n167 = Unbundle By Name(w452) -> ("DTU1_Common-Array_Q"=w451:refnum<queue>[], "DTU1_Common-Array_N"=w450:refnum<notifier>[], "DTU1_Combined-Array_Q"=w449:refnum<queue>[], "DTU1_Combined-Array_N"=w448:refnum<notifier>[], "DTU2_Combined-Array_Q"=w447:refnum<queue>[], "DTU2_Combined-Array_N"=w446:refnum<notifier>[])
        n168 = for {
          shift-right: [w474] -> w439
          shift-left: w445 -> [w480]
          tunnel: w451 -> [w478] mode=indexing
          tunnel: w450 -> [w477] mode=indexing
          shift-right: [w473] -> w438
          shift-left: w445 -> [w475]
          n169 = Release Queue(queue=w478, error in (no error)=w480) -> (error out=w479:errorcluster)  [unwired: 1 in, 2 out]
          n170 = Release Notifier(notifier=w477, error in (no error)=w475) -> (error out=w476:errorcluster)  [unwired: 1 in, 2 out]
          n171 = call <vilib>:"Clear Errors.vi"("error in (no error)"=w479) -> ("error out"=w474:errorcluster)  [unwired: 5 in, 1 out]
          n172 = call <vilib>:"Clear Errors.vi"("error in (no error)"=w476) -> ("error out"=w473:errorcluster)  [unwired: 5 in, 1 out]
        }
        n173 = for {
          shift-right: [w466] -> w441
          shift-left: w445 -> [w472]
          tunnel: w449 -> [w470] mode=indexing
          tunnel: w448 -> [w469] mode=indexing
          shift-right: [w465] -> w442
          shift-left: w445 -> [w467]
          n174 = Release Queue(queue=w470, error in (no error)=w472) -> (error out=w471:errorcluster)  [unwired: 1 in, 2 out]
          n175 = Release Notifier(notifier=w469, error in (no error)=w467) -> (error out=w468:errorcluster)  [unwired: 1 in, 2 out]
          n176 = call <vilib>:"Clear Errors.vi"("error in (no error)"=w471) -> ("error out"=w466:errorcluster)  [unwired: 5 in, 1 out]
          n177 = call <vilib>:"Clear Errors.vi"("error in (no error)"=w468) -> ("error out"=w465:errorcluster)  [unwired: 5 in, 1 out]
        }
        n178 = for {
          shift-right: [w458] -> w443
          shift-left: w445 -> [w464]
          tunnel: w447 -> [w462] mode=indexing
          tunnel: w446 -> [w461] mode=indexing
          shift-right: [w457] -> w444
          shift-left: w445 -> [w459]
          n179 = Release Queue(queue=w462, error in (no error)=w464) -> (error out=w463:errorcluster)  [unwired: 1 in, 2 out]
          n180 = Release Notifier(notifier=w461, error in (no error)=w459) -> (error out=w460:errorcluster)  [unwired: 1 in, 2 out]
          n181 = call <vilib>:"Clear Errors.vi"("error in (no error)"=w463) -> ("error out"=w458:errorcluster)  [unwired: 5 in, 1 out]
          n182 = call <vilib>:"Clear Errors.vi"("error in (no error)"=w460) -> ("error out"=w457:errorcluster)  [unwired: 5 in, 1 out]
        }
        n183 = Merge Errors(w439, w438, w441, w442, w443, w445, w444) -> (w454:errorcluster)
        n184 = call <vilib>:"Clear Errors.vi"("error in (no error)"=w454) -> ("error out"=w440:errorcluster)  [unwired: 5 in, 1 out]
        n185 = call "Enque_Message_FGV.vi"("Priority"=TRUE ("Priority Message? (F)"), "error in (no error)"=w440, "Message"="Exit") -> ("error out"=w453:errorcluster)  [unwired: 8 in]
      }
      frame "Exit" {
        # "Stop the VI"
        # "Release the message queue reference"
        # "#CodeNeeded - Add any required cleanup code here. Note that if 'Exit' was called as a result of an error, an error dialog will be displayed. Add any custom error handling for an 'Exit' condition here as well."
        # "Exit - Exit the application."
        n186 = disable-structure shown="Disabled" {
          disable-tunnel: w491 -> [w496 _]
          frame Disabled {
            n187 = Variant To Data(type=errorcluster {"status"=FALSE, "code"=0, "source"=""} ("error constant"), Variant=w496) -> (data=w497:errorcluster)  [unwired: 1 in, 1 out]
            n188 = call <vilib>:"Simple Error Handler.vi"("error in (no error)"=w497) -> ()  [unwired: 4 in, 5 out]
          }
          frame Enabled {
          }
        }
        n189 = call "Enque_Message_FGV.vi"("Priority"=TRUE ("Priority Message? (F)"), "error in (no error)"=w484, "Message"="Exit") -> ("error out"=w483:errorcluster)  [unwired: 8 in]
        n190 = call <vilib>:"Clear Errors.vi"("error in (no error)"=w483) -> ("error out"=w482:errorcluster)  [unwired: 5 in, 1 out]
        n191 = call "Fire User Event - Stop.vi"("User Event - Stop"=w488) -> ("error out"=w486:errorcluster)  [unwired: 10 in]
        n192 = call "Queue_Comm_FGV.vi"("error in (no error)"=w482, "Enum"=FGV_Queue_Control."Release") -> ("error Out"=w489:errorcluster)  [unwired: 8 in, 1 out]
        n193 = call "Fire User Event - Stop.vi"("User Event - Stop"=w492) -> ("error out"=w487:errorcluster)  [unwired: 10 in]
        n194 = Merge Errors(w487, w486, w489) -> (w493:errorcluster)
      }
      frame Default {
        # "'Default' case only runs if there is a message that isn't defined in any of the other cases.  Output a programming error."
        n195 = xnode "Error Ring"("parameter 0"=w499) -> ("error out"=w500:errorcluster)
      }
    }
    n196 = call "Error_Handler_MHL_FGV.vi"("error in (no error)"=w33) -> ("error Out"=w32:errorcluster)  [unwired: 10 in]
  }
  n197 = while {
    shift-right: [w512] -> w24
    shift-left: w21 -> [w513]
    tunnel: [w509] -> w22
    stop <- w511 stop-if-true
    # "Event Handling Loop"
    n198 = event shown="[4] \"FCT_Relay - OUTPUT\": Value Change" {
      selector: w513 -> [_ _ _ _ _ _ _ _ _]
      dyn-events: [_ _ _ _ _ _ _ _ _] -> w512
      timeout: _ -> [_ _ _ _ _ _ _ _ _]
      tunnel: [_ _ _ _ _ _ _ _ TRUE ("Discard?")] -> w511
      tunnel: [w515 w520 w522 w527 w531 w537 _ w541 _] -> w510
      event "Init. INSTR.": Value Change {
        n199 = event-data() -> ()  [unwired: 1 in, 1 out]
        n200 = call "Enque_Message_FGV.vi"("Priority"=TRUE ("Priority Message? (F)"), "Message"="Init_Inst") -> ("error out"=w515:errorcluster)  [unwired: 9 in]
      }
      event "FCT/EOL": Value Change {
        n201 = event-data() -> ()  [unwired: 1 in, 2 out]
        n202 = To Variant(anything="FCT/EOL") -> (Variant=w517:variant)
        n203 = call "Enque_Message_FGV.vi"("Message Data"=w517, "Message"="Init_Inst" ("Initial Message")) -> ("error out"=w520:errorcluster)  [unwired: 9 in]
      }
      event "DUT": Value Change {
        n204 = event-data() -> ()  [unwired: 1 in, 2 out]
        n205 = To Variant(anything="DUT") -> (Variant=w523:variant)
        n206 = call "Enque_Message_FGV.vi"("Message Data"=w523, "Message"="DUT" ("Initial Message")) -> ("error out"=w522:errorcluster)  [unwired: 9 in]
      }
      event Value Change {
        n207 = event-data() -> ()  [unwired: 1 in, 1 out]
        n208 = To Variant(anything="EOL_Relay - OUTPUT") -> (Variant=w526:variant)
        n209 = call "Enque_Message_FGV.vi"("Priority"=TRUE ("Priority Message? (F)"), "Message Data"=w526, "Message"="Digital output") -> ("error out"=w527:errorcluster)  [unwired: 8 in]
      }
      event Value Change {
        n210 = event-data() -> ()  [unwired: 1 in, 1 out]
        n211 = To Variant(anything="FCT_Relay - OUTPUT") -> (Variant=w532:variant)
        n212 = call "Enque_Message_FGV.vi"("Priority"=TRUE ("Priority Message? (F)"), "Message Data"=w532, "Message"="Digital output") -> ("error out"=w531:errorcluster)  [unwired: 8 in]
      }
      event Panel Close? {
        # "Send the 'Confirm Quit' message if the user closes the panel of the VI. Discard the event so the 'Confirm Quit' message has a chance to run."
        n213 = event-data() -> ()  [unwired: 1 in, 1 out]
        n214 = call "Enque_Message_FGV.vi"("Priority"=TRUE ("Priority Message? (F)"), "Message"="Confirm Quit") -> ("error out"=w537:errorcluster)  [unwired: 9 in]
        n215 = event-data("Discard?"=TRUE) -> ()  [unwired: 1 in, 1 out]
      }
      event Application Instance Close {
        # "#CodeRecommended - When a project closes, all VIs within that project are aborted and leave memory. However, any code placed in this event frame is guaranteed to run to completion, so add any cleanup code that absolutely must happen here."
        n216 = event-data() -> ()  [unwired: 1 in, 1 out]
      }
      event "Exit": Value Change {
        n217 = event-data() -> ()  [unwired: 1 in, 1 out]
        n218 = call "Enque_Message_FGV.vi"("Priority"=TRUE ("Priority Message? (F)"), "Message"="Confirm Quit") -> ("error out"=w541:errorcluster)  [unwired: 9 in]
      }
      event User Event {
        # "The Message Handling Loop processed an \"Exit\" message, which fired this event to stop the Event Handling Loop."
        n219 = event-data() -> ()  [unwired: 1 in, 1 out]
        n220 = local write "Display <Replace Me>"("\"Exit\" button pressed" ("VI Stopped")) -> ()
      }
    }
    n221 = call "Error_Handler_EHL_FGV.vi"("error in (no error)"=w510) -> ("error Out"=w509:errorcluster)  [unwired: 10 in]
  }
  n222 = while {
    shift-right: [w550] -> _
    shift-left: w6 -> [w548]
    shift-right: [w552] -> w4
    shift-left: w5 -> [w551]
    stop <- w544 stop-if-true
    n223 = Dequeue Element(queue=w548, error in (no error)=w551) -> (element=w547:T8, error out=w549:errorcluster)  [unwired: 1 in, 2 out]
    n224 = Unbundle(w547) -> ("Message"=w546:string, "Message Data"=w545:variant)
    n225 = case shown="\"Read_DI\", Default" w546 {
      tunnel: w548 -> [w554 w564 w567]
      tunnel: [w557 w565 w568] -> w552
      tunnel: w549 -> [w561 w566 w568]
      tunnel: [w554 w564 w567] -> w550
      tunnel: w545 -> [_ _ _]
      tunnel: [_ TRUE _] -> w544
      frame "Read_DI", Default {
        w562 = T11[] [enum."EMERGENCY", enum."CONTROL ON", enum."START DUT 1", enum."START DUT 2", enum."STOP DUT 1", enum."STOP DUT 2", enum."PPS DUT 1", enum."PPS DUT 2", enum."REED CYL UP DUT 1", enum."REED CYL DOWN DUT 1", enum."REED CYL UP DUT 2", enum."REED CYL DOWN DUT 2", enum."LIGHT CURTAIN"] items=["EMERGENCY", "CONTROL ON", "START DUT 1", "START DUT 2", "STOP DUT 1", "STOP DUT 2", "PPS DUT 1", "PPS DUT 2", "REED CYL UP DUT 1", "REED CYL DOWN DUT 1", "REED CYL UP DUT 2", "REED CYL DOWN DUT 2", "LIGHT CURTAIN"] ("PLC_BOOL_IN")
        n226 = call "MAP_FGV_IN.vi"("error in (no error)"=w561, "Relay_ENUM_IN"=w562) -> ("error out"=w560:errorcluster, "DOs_out"=w559:bool[])  [unwired: 7 in, 1 out]
        n227 = Array To Cluster(array=w559) -> (cluster=→"ADAM_Card - INPUT":T12)
        n228 = Bundle(cluster=T8 {"Message"="", "Message Data"=variant} ("element"), "Message"="Read_DI") -> (w553:T8)  [unwired: 1 in]
        n229 = Enqueue Element(queue=w554, element=w553, error in (no error)=w560) -> (error out=w557:errorcluster)  [unwired: 1 in, 2 out]
      }
      frame "Exit" {
        n230 = Release Queue(queue=w564, error in (no error)=w566) -> (error out=w565:errorcluster)  [unwired: 1 in, 2 out]
      }
      frame "Initialize" {
      }
    }
  }
  n231 = Unregister For Events(event registration refnum=w24, error in=w22) -> (error out=w25:errorcluster)
  n232 = Merge Errors(w25, w28, w4) -> (w26:errorcluster)
  n233 = call "Destroy User Event - Stop.vi"("error in (no error)"=w26, "User Event - Stop"=w7) -> ("error out"=w15:errorcluster)  [unwired: 9 in]
  n234 = call <vilib>:"Clear Errors.vi"("error in (no error)"=w15) -> ("error out"=w3:errorcluster)  [unwired: 5 in, 1 out]
  n235 = control-ref of="This VI"() -> (w2:refnum<vi>)
  n236 = invoke class="VI" method="FP.Close"(reference=w2, error in=w3) -> (error out=→"error in (out)":errorcluster)  [unwired: 1 in, 2 out]
